vi "Build Minor Frame Messages.vi"(7 "Virtual Memory Unit in":refnum<class "Virtual Memory Unit.lvclass">, 8 "error in (no error)":errorcluster, 10 "Starting Address":u16 format="%04x", 11 "Minor Frame in":refnum<class "Minor Frame.lvclass">) -> (0 "error out":errorcluster, 1 "Next Available Cmd Address":u16 format="%04x", 2 "Next Available Data Address":u16 format="%04x", 3 "Minor Frame out":refnum<class "Minor Frame.lvclass">, 5 "Virtual Memory Unit out":refnum<class "Virtual Memory Unit.lvclass">)   [LabVIEW 2020, in "BCI-1553 API.lvlib" / "Minor Frame.lvclass"]
doc: "Very closely resembles the Major Frame scheduling. Retrieves a message off of the schedule queue and\nthen checks to see if any of the messages have a matching ID. If the ID matches, the message is placed\ninto the instruction list for this minor frame subroutine. Additionally, the configuration and data for the\nmessage is constructed. This requires a prediction of the length of the minor frame."
uses:
  Minor Frame.lvclass
  Dependencies/Virtual Memory Unit/Virtual Memory Unit.lvclass
  Minor Frame.lvclass/Minor Frame.ctl
  TypeDefs/Message Pointers.ctl
  BCI-1553 API.lvlib
  Message/Message.lvclass
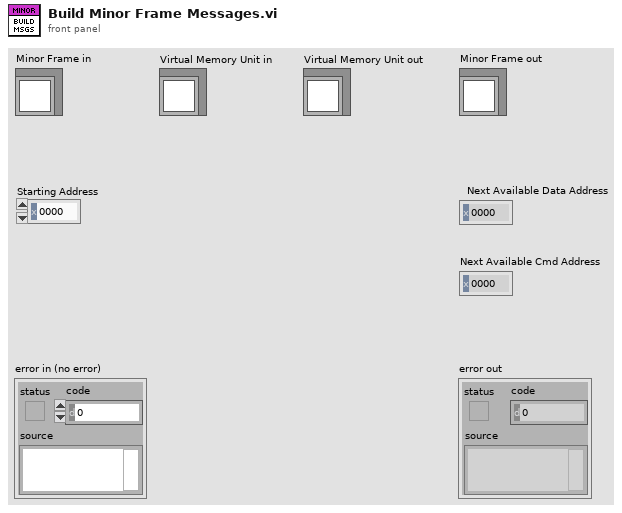
[diagram p1: front panel]
types:
  T1 = typedef "BCI-1553 API.lvlib/Message Pointers.ctl" = cluster{"SubRoutine Address":u16, "HP Async Address":u16}
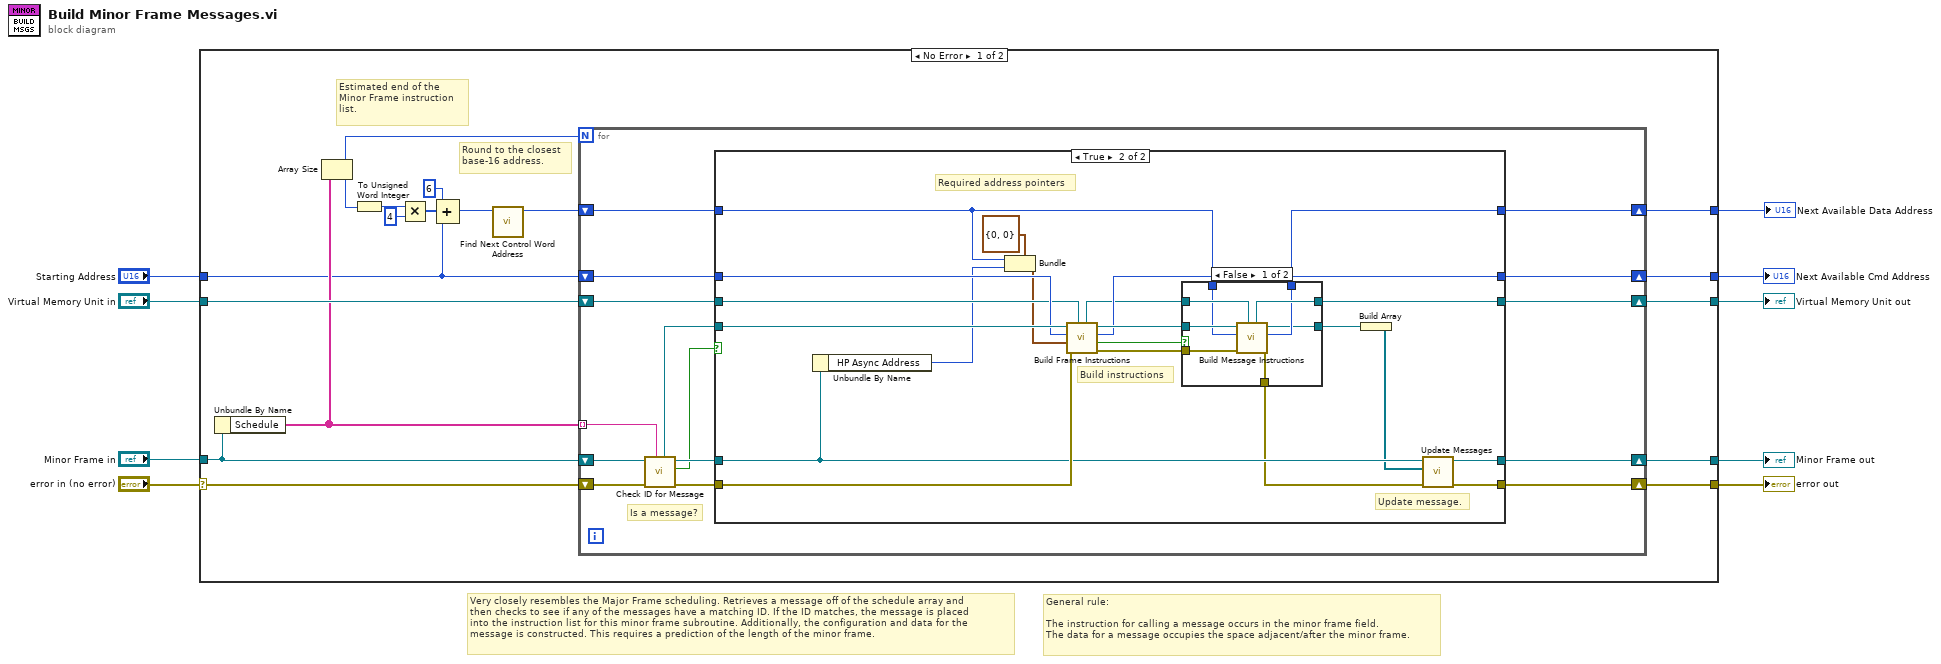
[diagram p0: block diagram]
diagram:
  # "General rule:\n\nThe instruction for calling a message occurs in the minor frame field.\nThe data for a message occupies the space adjacent/after the minor frame."
  # "Very closely resembles the Major Frame scheduling. Retrieves a message off of the schedule array and\nthen checks to see if any of the messages have a matching ID. If the ID matches, the message is placed\ninto the instruction list for this minor frame subroutine. Additionally, the configuration and data for the\nmessage is constructed. This requires a prediction of the length of the minor frame."
  n1 = case shown="No Error" "error in (no error)" {
    selector: "error in (no error)" -> [w24 w83]
    tunnel: [w23 w83] -> w8
    tunnel: [w25 w82] -> w6
    tunnel: "Minor Frame in" -> [w26 w82]
    tunnel: "Virtual Memory Unit in" -> [w21 w81]
    tunnel: "Starting Address" -> [w12 w80]
    tunnel: [w20 w81] -> w3
    tunnel: [w22 w80] -> w2
    tunnel: [w10 _] -> w1
    frame No Error {
      # "Round to the closest\nbase-16 address."
      # "Estimated end of the\nMinor Frame instruction\nlist."
      n2 = Unbundle By Name(w26) -> ("Schedule"=w14:string[])
      n3 = Array Size(array=w14) -> (size(s)=w11:i32)
      n4 = To Unsigned Word Integer(number=w11) -> (unsigned 16bit integer=w15:u16)
      n5 = Multiply(x=w15, y=u16 4) -> (x*y=w17:u16)
      n6 = Compound Arithmetic op=ADD(u16 6 ("value"), w17, w12) -> (w19:u16)
      n7 = call "Find Next Control Word Address.vi"("Starting Address"=w19) -> ("0xHHHX Address"=w13:u16)  [unwired: 10 in]
      n8 = for {
        N: w11 -> [_]
        shift-right: [w39] -> w25
        shift-left: w26 -> [w40]
        shift-right: [w41] -> w23
        shift-left: w24 -> [w31]
        shift-right: [w35] -> w22
        shift-left: w12 -> [w37]
        shift-right: [w34] -> w20
        shift-left: w21 -> [w38]
        tunnel: w14 -> [w32] mode=indexing
        shift-right: [w33] -> w10
        shift-left: w13 -> [w36]
        # "Is a message?"
        n9 = call "Check ID for Message.vi"("ID"=w32, "error in (no error)"=w31, "Minor Frame in"=w40) -> ("error out"=w29:errorcluster, "Msg Found?"=w27:bool, "Minor Frame out"=w30:refnum<class "Minor Frame.lvclass">, "Message"=w28:refnum<class "Message.lvclass">)  [unwired: 5 in]
        n10 = case shown="True" w27 {
          tunnel: w28 -> [_ w67]
          tunnel: w29 -> [w43 w64]
          tunnel: [w43 w49] -> w41
          tunnel: w38 -> [w44 w61]
          tunnel: [w44 w59] -> w34
          tunnel: [w45 w62] -> w35
          tunnel: w37 -> [w45 w63]
          tunnel: [w46 w58] -> w33
          tunnel: w36 -> [w46 w55]
          tunnel: w30 -> [w42 w53]
          tunnel: [w42 w52] -> w39
          frame False {
            # "Not a message"
          }
          frame True {
            # "Required address pointers"
            # "Update message."
            # "Build instructions"
            n11 = Unbundle By Name(w53) -> ("HP Async Address"=w48:u16)
            n12 = Bundle(cluster=T1 {"SubRoutine Address"=0, "HP Async Address"=0} ("Message Pointers"), "SubRoutine Address"=w55, "HP Async Address"=w48) -> (w54:T1)
            n13 = call "Build Frame Instructions.vi"("Virtual Memory Unit in"=w61, "error in (no error)"=w64, "Message Pointers"=w54, "Starting Address"=w63, "Message in"=w67) -> ("error out"=w65:errorcluster, "Msg Already Configured"=w47:bool, "Next Available Address"=w62:u16, "Message out"=w66:refnum<class "Message.lvclass">, "Virtual Memory Unit out"=w60:refnum<class "Virtual Memory Unit.lvclass">)  [unwired: 2 in]
            n14 = case shown="False" w47 {
              tunnel: w66 -> [w75 w77]
              tunnel: w65 -> [w74 w76]
              tunnel: w60 -> [w73 w79]
              tunnel: [w72 w79] -> w59
              tunnel: [w71 w78] -> w58
              tunnel: [w70 w77] -> w57
              tunnel: w55 -> [w69 w78]
              tunnel: [w68 w76] -> w50
              frame False {
                n15 = call "Build Message Instructions.vi"("Virtual Memory Unit in"=w73, "error in (no error)"=w74, "Starting Address"=w69, "Message in"=w75) -> ("error out"=w68:errorcluster, "Next Available Address"=w71:u16, "Message out"=w70:refnum<class "Message.lvclass">, "Virtual Memory Unit out"=w72:refnum<class "Virtual Memory Unit.lvclass">)  [unwired: 4 in]
              }
              frame True {
              }
            }
            n16 = Build Array(w57) -> (w51:refnum<class "Message.lvclass">[])
            n17 = call "Update Messages.vi"("error in (no error)"=w50, "Messages"=w51, "Minor Frame in"=w53) -> ("error out"=w49:errorcluster, "Minor Frame out"=w52:refnum<class "Minor Frame.lvclass">)  [unwired: 7 in]
          }
        }
      }
    }
    frame Error {
    }
  }
  "error out" <- w8
  "Minor Frame out" <- w6
  "Virtual Memory Unit out" <- w3
  "Next Available Cmd Address" <- w2
  "Next Available Data Address" <- w1
